vi "Argparse Example.vi"() -> ()   [LabVIEW 2020]
uses:
  8d223fd8-e801-47c5-b941-cb57a943469c.vi
  LV-Argparse/LV ArgParse.lvlib
  LV-Argparse/LV Argument Parser/Argument Definition.ctl
  LV-Argparse/LV Argument Parser/LV Argument Parser.lvclass
  LV-Argparse/LV Argument Parser/Setup.vi
  LV-Argparse/LV Argument Parser/Parse.vi
  LV-Argparse/LV Argument Parser/Obtain.vi
  LV-Argparse/LV Argument Parser/Fill VCluster.vi
  LV-Argparse/LV Argument Parser/Get Argument.vi
  LV-Argparse/LV Argument Parser/Get Path.vi
panel:
  out "data":T1
  out "Output":string
  out "Config Path":path
  out "error out":errorcluster
  out "numbers":i32[](array[numeric])
  out "Parsed Data":map{string, variant[]}(c390)
  out "Message":string
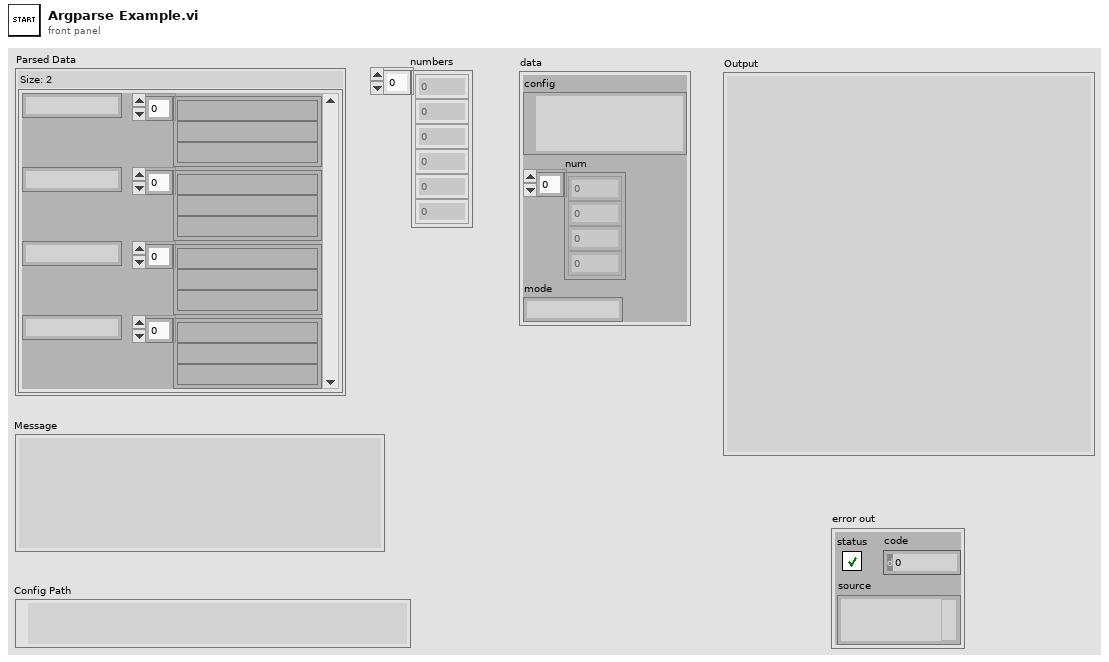
[diagram p1: front panel]
types:
  T1 = cluster{"config":path, "num":i32[], "mode":string}
  T2 = typedef "LV ArgParse.lvlib/LV Argument Parser.lvclass/Argument Definition.ctl" = cluster{"Name":string, "short (positional)":string, "long (positional)":string, "action":enum16{"store", "store-const", "store-false", "store-true", "append", "append-const", "count", "help", "version"}, "choices":string[], "const":string, "default":string, "dest (=name)":string, "help":string, "Number":i32, "Required":bool, "Type":enum16{"String", "Int", "UInt", "Float", "Bool", "Date", "Path"}}
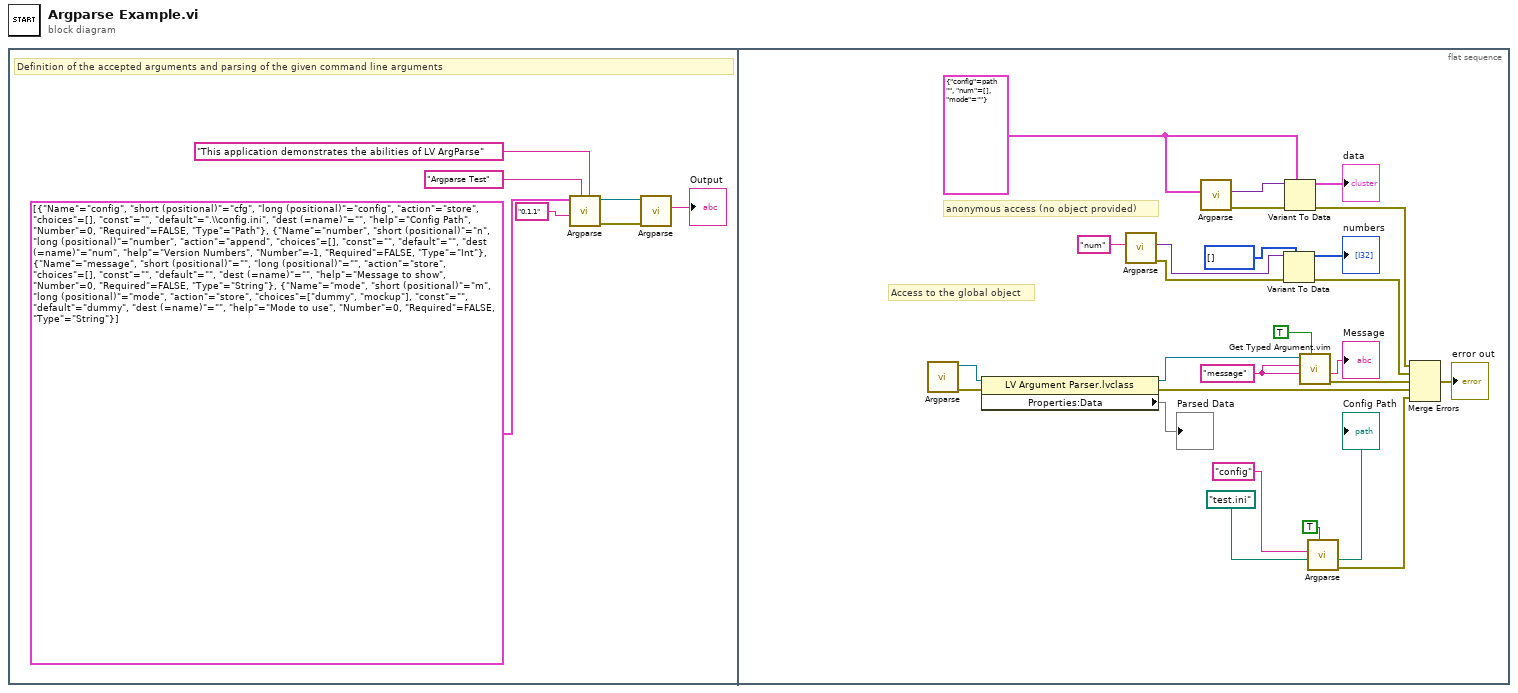
[diagram p0: block diagram]
diagram:
  n1 = flat-sequence {
    frame #0 {
      # "Definition of the accepted arguments and parsing of the given command line arguments"
      n2 = call-poly "Argparse.vi"("Description"="This application demonstrates the abilities of LV ArgParse", "Name"="Argparse Test", "Version"="0.1.1", "Arguments"=T2[] [{"Name"="config", "short (positional)"="cfg", "long (positional)"="config", "action"=enum."store", "choices"=[], "const"="", "default"=".\\config.ini", "dest (=name)"="", "help"="Config Path", "Number"=0, "Required"=FALSE, "Type"=enum."Path"}, {"Name"="number", "short (positional)"="n", "long (positional)"="number", "action"=enum."append", "choices"=[], "const"="", "default"="", "dest (=name)"="num", "help"="Version Numbers", "Number"=-1, "Required"=FALSE, "Type"=enum."Int"}, {"Name"="message", "short (positional)"="", "long (positional)"="", "action"=enum."store", "choices"=[], "const"="", "default"="", "dest (=name)"="", "help"="Message to show", "Number"=0, "Required"=FALSE, "Type"=enum."String"}, {"Name"="mode", "short (positional)"="m", "long (positional)"="mode", "action"=enum."store", "choices"=["dummy", "mockup"], "const"="", "default"="dummy", "dest (=name)"="", "help"="Mode to use", "Number"=0, "Required"=FALSE, "Type"=enum."String"}]) -> ("error out"=w2:errorcluster, "LV Argument Parser out"=w7:refnum<class "LV Argument Parser.lvclass">)  [unwired: 6 in]
      n3 = call-poly "Argparse.vi"("error in (no error)"=w2, "LV Argument Parser in (Global)"=w7) -> ("Output"=→"Output":string)  [unwired: 7 in, 2 out]
    }
    frame #1 {
      w22 = T1 {"config"=path "", "num"=[], "mode"=""}
      w33 = "message" ("Name")
      # "anonymous access (no object provided)"
      # "Access to the global object"
      n4 = call-poly "Argparse.vi"() -> ("error out"=w30:errorcluster, "LV Argument Parser out"=w31:refnum<class "LV Argument Parser.lvclass">)  [unwired: 10 in]
      n5 = property class="LV Argument Parser.lvclass"(reference=w31, error in=w30) -> (reference out=w29:refnum<class "LV Argument Parser.lvclass">, error out=w26:errorcluster, "Properties:Data"=→"Parsed Data":map{string, variant[]})
      n6 = call-poly "Argparse.vi"("Name"="num") -> ("error out"=w18:errorcluster, "element"=w17:variant)  [unwired: 7 in, 2 out]
      n7 = call-poly "Argparse.vi"("Cluster In"=w22) -> ("error out"=w20:errorcluster, "Filled Cluster Out"=w21:variant)  [unwired: 8 in, 1 out]
      n8 = Variant To Data(error in=w18, type=i32[] [], Variant=w17) -> (data=→"numbers":i32[], error out=w14:errorcluster)
      n9 = Variant To Data(error in=w20, type=w22, Variant=w21) -> (data=→"data":T1, error out=w13:errorcluster)
      n10 = call "Get Typed Argument.vim"("Optional (F)"=TRUE, "Type / Default"=w33, "Name"=w33, "LV Argument Parser in (global)"=w29) -> ("error out"=w27:errorcluster, "data"=→"Message":string)  [unwired: 4 in, 2 out]
      n11 = call-poly "Argparse.vi"("Optional"=TRUE, "Default"=path "test.ini", "Name"="config") -> ("error out"=w9:errorcluster, "Value"=→"Config Path":path)  [unwired: 5 in, 2 out]
      n12 = Merge Errors(w13, w14, w27, w26, w9) -> (→"error out":errorcluster)
    }
  }
